vi "TSPopup.Position Cluster.vi"(8 "error in (no error)":errorcluster, 10 "Mouse Coords":cluster{"x":i32, "y":i32}, 11 "Ctl Refnum":refnum<vi>) -> (0 "error out":errorcluster, 2 "Cluster Pos":cluster{"x":i32, "y":i32}, 3 "dup ref":refnum<vi>)   [LabVIEW 2016, in "TSPopup.lvlib" / "TSPopup.lvclass"]
doc: "Sets the position of the popup controls that are clusters (with OK and Cancel buttons).\n\nType Sensitive Popup \nCopyright © 2007, J. David Saunders\nAll rights reserved."
uses:
  <userlib>/TSPopup/TSPopup.lvclass
panel:
  # "Type Sensitive Popup \nCopyright © 2007, J. David Saunders\nAll rights reserved."
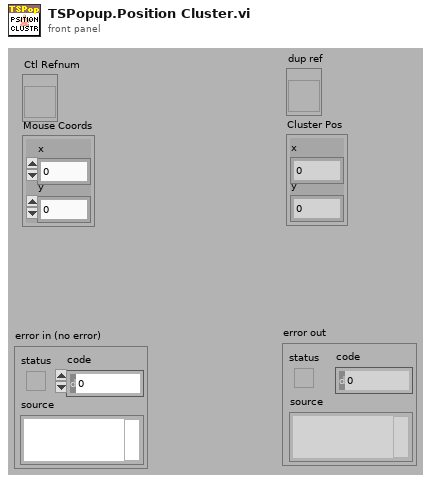
[diagram p1: front panel]
types:
  T1 = enum16{"right/low", "right/high", "left/low", "left/high", "Center"}
  T2 = typedef "LVRectTypeDef.ctl" = cluster{"Left":i16, "Top":i16, "Right":i16, "Bottom":i16}
  T3 = typedef "LVBoundsTypeDef.ctl" = cluster{"Width":u32, "Height":u32}
  T4 = typedef "LVPointTypeDef.ctl" = cluster{"Horizontal":i16, "Vertical":i16}
  T5 = cluster{"Left":i32, "Top":i32, "Right":i32, "Bottom":i32}
  T6 = cluster{"left":i16, "top":i16, "right":i16, "bottom":i16}
  T7 = cluster{"left":i32, "top":i32, "right":i32, "bottom":i32}
  T8 = cluster{"left":i32, "top":i32, "left":i32, "top":i32}
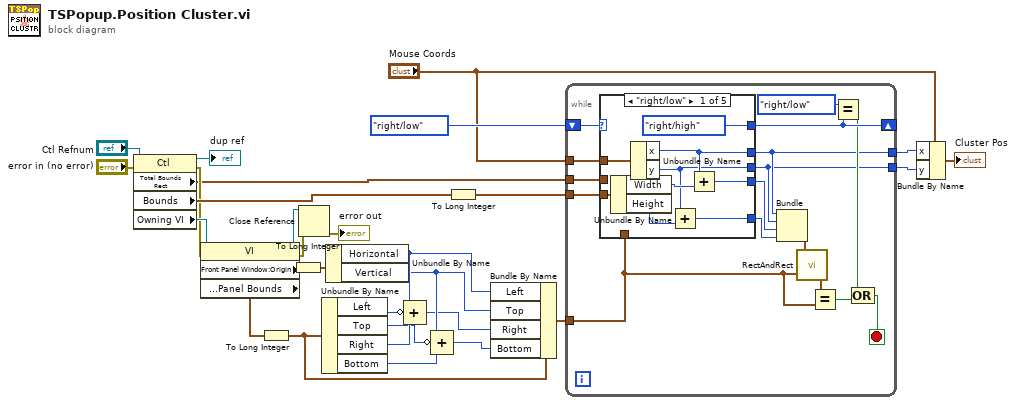
[diagram p0: block diagram]
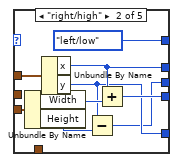
[diagram p2: hidden frame]
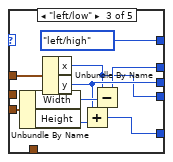
[diagram p3: hidden frame]
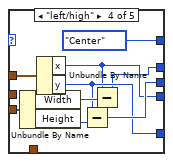
[diagram p4: hidden frame]
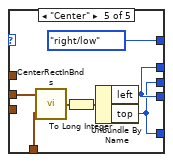
[diagram p5: hidden frame]
diagram:
  n1 = property class="Ctl"(reference="Ctl Refnum", error in="error in (no error)") -> (reference out=→"dup ref":refnum<vi>, error out=w9:errorcluster, "Total Bounds Rect"=w8:T2, "Bounds"=w25:T3, "Owning VI"=w17:refnum<vi>)
  n2 = property class="VI"(reference=w17, error in=w9) -> (reference out=w16:refnum<vi>, error out=w15:errorcluster, "Front Panel Window:Origin"=w28:T4, "Front Panel Window:Panel Bounds"=w3:T2)
  n3 = To Long Integer(number=w3) -> (32bit integer=w2:T5)
  n4 = To Long Integer(number=w28) -> (32bit integer=w10:cluster{"Horizontal":i32, "Vertical":i32})
  n5 = Close Reference(reference=w16, error in (no error)=w15) -> (error out=→"error out":errorcluster)
  n6 = Unbundle By Name(w2) -> ("Left"=w27:i32, "Top"=w11:i32, "Right"=w22:i32, "Bottom"=w26:i32)
  n7 = Unbundle By Name(w10) -> ("Horizontal"=w7:i32, "Vertical"=w6:i32)
  n8 = Compound Arithmetic op=ADD(w7, invert w27, w22) -> (w5:i32)
  n9 = Compound Arithmetic op=ADD(w6, invert w11, w26) -> (w4:i32)
  n10 = To Long Integer(number=w25) -> (32bit integer=w23:cluster{"Width":i32, "Height":i32})
  n11 = Bundle By Name(cluster=w2, "Left"=w7, "Top"=w6, "Right"=w5, "Bottom"=w4) -> (w1:T5)
  n12 = while {
    tunnel: w23 -> [w45]
    shift-right: [w42] -> _
    shift-left: T1."right/low" -> [w44]
    tunnel: "Mouse Coords" -> [w43]
    tunnel: [w37] -> w21
    tunnel: [w36] -> w20
    tunnel: w8 -> [w38]
    tunnel: w1 -> [w31]
    stop <- w40 stop-if-true
    n13 = case shown="\"right/low\"" w44 {
      tunnel: w45 -> [w53 w62 w71 w80 _]
      tunnel: w43 -> [w54 w63 w72 w81 _]
      tunnel: [T1."right/high" T1."left/low" T1."left/high" T1."Center" T1."right/low"] -> w42
      tunnel: [w50 w59 w66 w74 w87] -> w37
      tunnel: [w49 w56 w68 w77 w86] -> w36
      tunnel: [w48 w58 w65 w75 w87] -> w35
      tunnel: [w47 w57 w67 w76 w86] -> w34
      tunnel: w31 -> [_ _ _ _ w83]
      tunnel: w38 -> [_ _ _ _ w84]
      frame "right/low" {
        n14 = Unbundle By Name(w53) -> ("Width"=w52:i32, "Height"=w51:i32)
        n15 = Unbundle By Name(w54) -> ("x"=w50:i32, "y"=w49:i32)
        n16 = Add(x=w49, y=w51) -> (x+y=w47:i32)
        n17 = Add(x=w50, y=w52) -> (x+y=w48:i32)
      }
      frame "right/high" {
        n18 = Unbundle By Name(w62) -> ("Width"=w61:i32, "Height"=w60:i32)
        n19 = Unbundle By Name(w63) -> ("x"=w59:i32, "y"=w57:i32)
        n20 = Subtract(x=w57, y=w60) -> (x-y=w56:i32)
        n21 = Add(x=w59, y=w61) -> (x+y=w58:i32)
      }
      frame "left/low" {
        n22 = Unbundle By Name(w71) -> ("Width"=w70:i32, "Height"=w69:i32)
        n23 = Unbundle By Name(w72) -> ("x"=w65:i32, "y"=w68:i32)
        n24 = Add(x=w68, y=w69) -> (x+y=w67:i32)
        n25 = Subtract(x=w65, y=w70) -> (x-y=w66:i32)
      }
      frame "left/high" {
        n26 = Unbundle By Name(w80) -> ("Width"=w79:i32, "Height"=w78:i32)
        n27 = Unbundle By Name(w81) -> ("x"=w75:i32, "y"=w76:i32)
        n28 = Subtract(x=w76, y=w78) -> (x-y=w77:i32)
        n29 = Subtract(x=w75, y=w79) -> (x-y=w74:i32)
      }
      frame "Center" {
        n30 = call <vilib>:"CenterRectInBnds.vi"("bounds"=w83, "rect"=w84) -> ("centered rect"=w82:T6)
        n31 = To Long Integer(number=w82) -> (32bit integer=w85:T7)
        n32 = Unbundle By Name(w85) -> ("left"=w87:i32, "top"=w86:i32)
      }
    }
    n33 = Bundle("left"=w37, "top"=w36, "left"=w35, "top"=w34) -> (w33:T8)  [unwired: 1 in]
    n34 = call <vilib>:"RectAndRect.vi"("rect b"=w31, "rect a"=w33) -> ("union rect"=w32:T6)
    n35 = Equal?(x=w32, y=w31) -> (x = y?=w30:bool)
    n36 = Equal?(x=T1."right/low", y=w42) -> (x = y?=w41:bool)
    n37 = Compound Arithmetic op=OR(w41, w30) -> (w40:bool)
  }
  n38 = Bundle By Name(cluster="Mouse Coords", "x"=w21, "y"=w20) -> (→"Cluster Pos":cluster{"x":i32, "y":i32})
